vi "Analysis.vi"(8 "error in":errorcluster, 10 "queue in":refnum<queue>, 11 "User Event in":refnum<user-event>) -> (0 "error out":errorcluster)   [LabVIEW 2016]
uses:
  DataEvent.ctl
  DataEvent/EventType.ctl
  Analysis/AnalysisEnum.ctl
  FGV/GetSetEnum.ctl
  <vilib>/measure/maspectr.llb/FFT Power Spectrum and PSD for 1 Chan.vi
  <vilib>/measure/NI_MAPro.lvlib
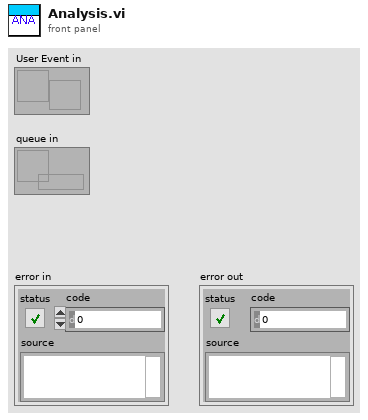
[diagram p1: front panel]
types:
  T1 = typedef "AnalysisEnum.ctl" = enum16{"Idle", "Analysis"}
  T2 = typedef "GetSetEnum.ctl" = enum16{"Get", "Set"}
  T3 = typedef "DataEvent.ctl" = cluster{"event type":T4, "data":variant}
  T4 = typedef "EventType.ctl" = enum16{"spectrum", "time", "exit"}
  T5 = typedef "ASIOData.ctl" = cluster{"Buffer Config":cluster{"# buffers":i32, "Buffer size":i32, "unit (ms)":enum16{"time (ms)", "Samples"}}, "Format (44kHz, 16Bit, stereo)":cluster{"Rate":i32, "Bits":i32, "Channels":u32}, "Play":bool, "Exit":bool}
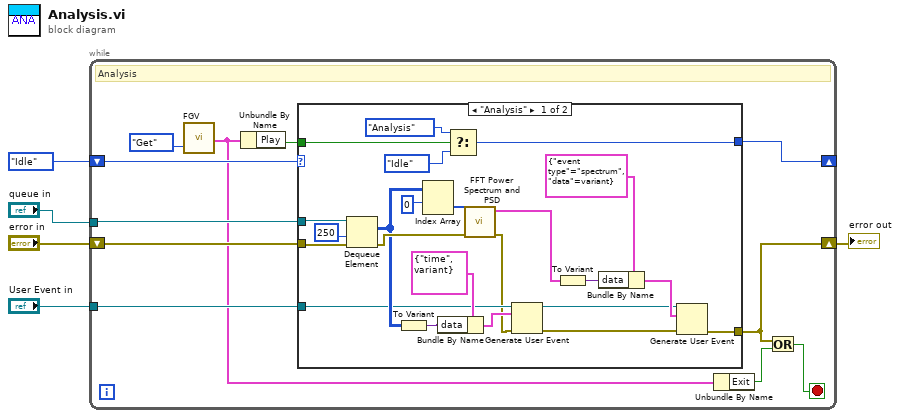
[diagram p0: block diagram]
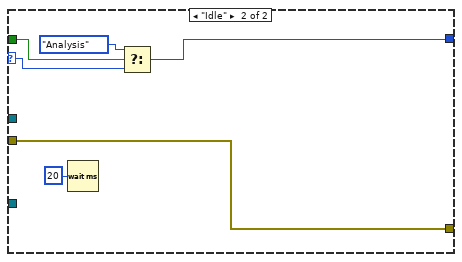
[diagram p2: hidden frame]
diagram:
  n1 = while {
    tunnel: "queue in" -> [w14]
    shift-right: [w11] -> _
    shift-left: AnalysisEnum."Idle" -> [w16]
    shift-right: [w10] -> w4
    shift-left: "error in" -> [w13]
    tunnel: "User Event in" -> [w8]
    stop <- w9 stop-if-true
    # "Analysis"
    n2 = call "FGV.vi"("GetSetEnum"=GetSetEnum."Get") -> ("ASIODataOut"=w7:T5)  [unwired: 1 in]
    n3 = Unbundle By Name(w7) -> ("Play"=w12:bool)
    n4 = case shown="\"Analysis\"" w16 {
      selector: w16 -> [_ w41]
      tunnel: w14 -> [w39 _]
      tunnel: w13 -> [w38 w43]
      tunnel: w12 -> [w18 w40]
      tunnel: [w35 w44] -> w11
      tunnel: [w19 w43] -> w10
      tunnel: w8 -> [w27 _]
      frame "Analysis" {
        n5 = Dequeue Element(queue=w39, timeout in ms (-1)=250, error in (no error)=w38) -> (element=w31:i32[][], error out=w34:errorcluster)  [unwired: 2 out]
        n6 = To Variant(anything=w31) -> (Variant=w29:variant)
        n7 = Index Array(array=w31, index (row)=0) -> (element=w32:i32[])  [unwired: 1 in]
        n8 = Bundle By Name(cluster=T3 {"event type"=enum."time", "data"=variant} ("data event"), "data"=w29) -> (w28:T3)
        n9 = Select(t=AnalysisEnum."Analysis", s=w18, f=AnalysisEnum."Idle") -> (s? t:f=w35:T1)
        n10 = call-poly <vilib>:"FFT Power Spectrum and PSD.vi"("error in (no error)"=w34, "time signal"=w32) -> ("error out"=w21:errorcluster, "Power Spectrum / PSD"=w22:cluster{"f0":dbl, "df":dbl, "magnitude":dbl[]})  [unwired: 6 in, 2 out]
        n11 = Generate User Event(user event=w27, event data cluster=w28, error in=w21) -> (user event out=w23:refnum<user-event>, error out=w20:errorcluster)  [unwired: 1 in]
        n12 = To Variant(anything=w22) -> (Variant=w25:variant)
        n13 = Bundle By Name(cluster=T3 {"event type"=enum."spectrum", "data"=variant} ("data event"), "data"=w25) -> (w26:T3)
        n14 = Generate User Event(user event=w23, event data cluster=w26, error in=w20) -> (error out=w19:errorcluster)  [unwired: 1 in, 1 out]
      }
      frame "Idle" {
        n15 = Wait (ms)(milliseconds to wait=u32 20) -> ()  [unwired: 1 out]
        n16 = Select(t=AnalysisEnum."Analysis", s=w40, f=w41) -> (s? t:f=w44:T1)
      }
    }
    n17 = Unbundle By Name(w7) -> ("Exit"=w6:bool)
    n18 = Or(x=w10, y=w6) -> (x .or. y?=w9:bool)
  }
  "error out" <- w4
